vi "Initialize Variables.vi"   [LabVIEW 2009]
uses:
  Functional Global Variables/Actions for FG's.ctl
  Intelligence/VFH/VFH Parameters.ctl
  Intelligence/VFH/VFH Weights.ctl
  TypeDefs/Queue TypeDefs/Motor Instruction.ctl
  TypeDefs/Queue TypeDefs/Motor State.ctl
  Remote Control/Motor Command.ctl
types:
  T1 = typedef "Actions for FG's.ctl" = enum16{"Read", "Write"}
  T2 = typedef "VFH Parameters.ctl" = cluster{"Robot Radius":u16, "Near Threshold":u16, "Mid Threshold":u16, "Far Threshold":u16, "Weights":T3}
  T3 = typedef "VFH Weights.ctl" = cluster{"TS-S weight":dbl, "CS-S weight":dbl, "PCS-S weight":dbl, "Near weight":dbl, "Mid weight":dbl, "Far weight":dbl}
  T4 = typedef "Motor Instruction.ctl" = cluster{"Motor State":T5, "Motor Command":T6}
  T5 = typedef "Motor State.ctl" = enum16{"Wait", "Initialize", "Check FET", "Run", "Stop"}
  T6 = typedef "Motor Command.ctl" = cluster{"Speed":i16, "Turn":i16}
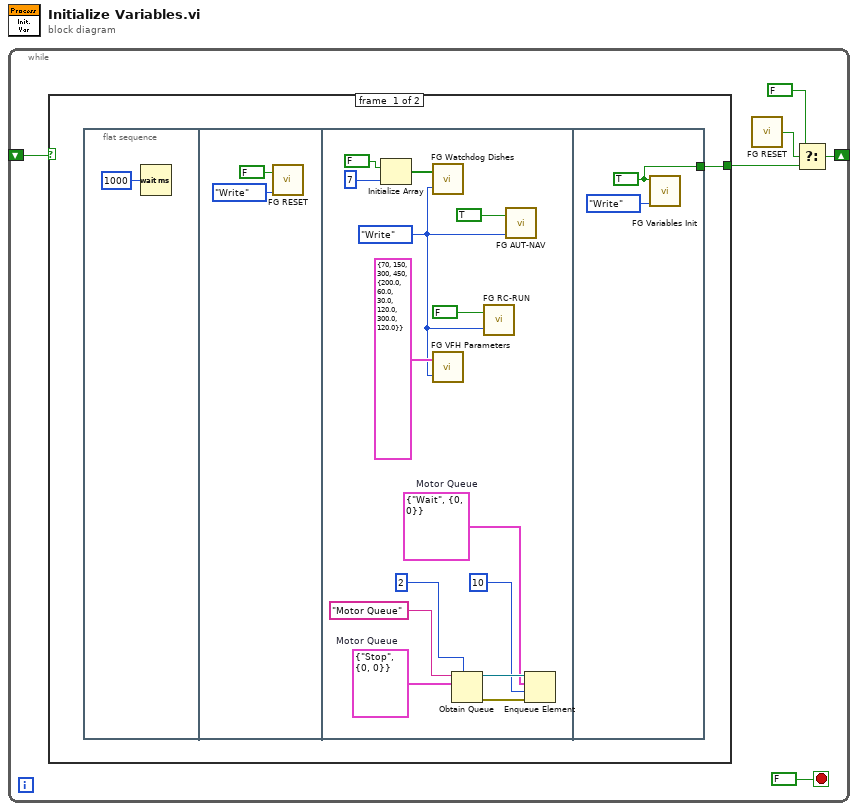
[diagram p0: block diagram]
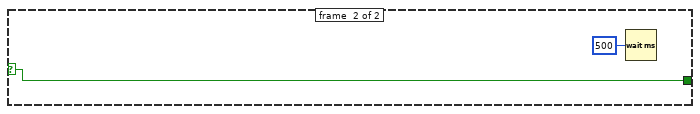
[diagram p2: hidden frame]
diagram:
  n1 = while {
    shift-right: [w4] -> _
    shift-left: _ -> [w3]
    stop <- FALSE stop-if-true
    n2 = case shown="False" w3 {
      selector: w3 -> [_ w28]
      tunnel: [w7 w28] -> w2
      frame #0 {
        n3 = flat-sequence {
          tunnel: [w25] -> w7
          frame #0 {
            n4 = Wait (ms)(milliseconds to wait=u32 1000) -> ()  [unwired: 1 out]
          }
          frame #1 {
            n5 = call "FG RESET.vi"("FG Action (Read)"=Actions_for_FG's."Write" ("FG Action"), "RESET in"=FALSE ("Variables Init in")) -> ()  [unwired: 1 out]
          }
          frame #2 {
            w19 = T4 {"Motor State"=enum."Wait", "Motor Command"={"Speed"=0, "Turn"=0}}  # Motor Queue
            w20 = T4 {"Motor State"=enum."Stop", "Motor Command"={"Speed"=0, "Turn"=0}}  # Motor Queue
            w12 = Actions_for_FG's."Write" ("FG Action")
            n6 = Initialize Array(FALSE ("Variables Init in"), 7 ("dimension size")) -> (w15:bool[])
            n7 = call "FG Watchdog Dishes.vi"("FG Action (Read)"=w12, "Watchdog dishes in"=w15) -> ()  [unwired: 1 out]
            n8 = call "FG VFH Parameters.vi"("FG Action (Read)"=w12, "VFH Parameters in"=T2 {"Robot Radius"=70, "Near Threshold"=150, "Mid Threshold"=300, "Far Threshold"=450, "Weights"={"TS-S weight"=200.0, "CS-S weight"=60.0, "PCS-S weight"=30.0, "Near weight"=120.0, "Mid weight"=300.0, "Far weight"=120.0}}) -> ()  [unwired: 1 in, 1 out]
            n9 = Obtain Queue(max queue size (-1, unlimited)=2, name (unnamed)="Motor Queue", element data type=w20) -> (queue out=w23:refnum<queue>, error out=w17:errorcluster)  [unwired: 2 in, 1 out]
            n10 = call "FG RC-RUN.vi"("FG Action (Read)"=w12, "RC/!Run in"=FALSE ("Run/RC")) -> ()  [unwired: 1 in, 1 out]
            n11 = call "FG AUT-NAV.vi"("FG Action (Read)"=w12, "Aut/!Nav in"=TRUE) -> ()  [unwired: 1 out]
            n12 = Enqueue Element(queue=w23, element=w19, timeout in ms (-1)=10, error in (no error)=w17) -> ()  [unwired: 3 out]
          }
          frame #3 {
            w25 = TRUE ("Variables Init in")
            n13 = call "FG Variables Init.vi"("FG Action"=Actions_for_FG's."Write", "Variables Init in"=w25) -> ()  [unwired: 9 in, 1 out]
          }
        }
      }
      frame #1 {
        n14 = Wait (ms)(milliseconds to wait=u32 500) -> ()  [unwired: 1 out]
      }
    }
    n15 = call "FG RESET.vi"() -> ("RESET out"=w6:bool)  [unwired: 2 in]
    n16 = Select(t=FALSE, s=w6, f=w2) -> (s? t:f=w4:bool)
  }
